vi "BilinearInterpolation.vi"(1 "Column Index":dbl, 2 "Row Index":dbl, 3 "Array":dbl[][](array[numeric])) -> (0 "Bilinear Interpolated Value":dbl)   [LabVIEW 2012]
uses:
  <vilib>/Analysis/baseanly.llb/Real Outer Product.vi
  <vilib>/Analysis/NI_AALBase.lvlib
panel:
  # "Bilinear Interpolation of a 2D array\n\n\nChristian Altenbach, June 2005\ncaltenba@ucla.edu"
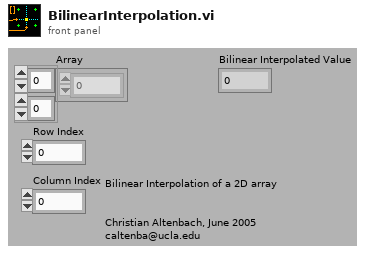
[diagram p1: front panel]
types:
  T1 = typedef "NI_Matrix.lvlib/RealMatrix.ctl" = dbl[][]
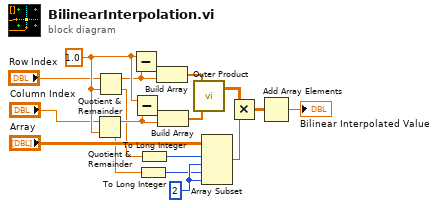
[diagram p0: block diagram]
diagram:
  w12 = 1.0 ("x")
  w18 = 2 ("length")
  n1 = Quotient & Remainder(x="Column Index", y=w12) -> (x-y*floor(x/y)=w7:dbl, floor(x/y)=w2:dbl)
  n2 = Quotient & Remainder(x="Row Index", y=w12) -> (x-y*floor(x/y)=w9:dbl, floor(x/y)=w3:dbl)
  n3 = Subtract(x=w12, y=w9) -> (x-y=w8:dbl)
  n4 = Subtract(x=w12, y=w7) -> (x-y=w6:dbl)
  n5 = To Long Integer(number=w2) -> (32bit integer=w14:i32)
  n6 = To Long Integer(number=w3) -> (32bit integer=w15:i32)
  n7 = Build Array(w8, w9) -> (w10:dbl[])
  n8 = Build Array(w6, w7) -> (w11:dbl[])
  n9 = call-poly <vilib>:"Outer Product.vi"("Y Vector"=w11, "X Vector"=w10) -> ("Outer Product"=w1:T1)  [unwired: 1 out]
  n10 = Array Subset(array="Array", index (row)=w15, length (row)=w18, index (col)=w14, length (col)=w18) -> (w13:dbl[][])
  n11 = Multiply(x=w1, y=w13) -> (x*y=w16:T1)
  n12 = Add Array Elements(numeric array=w16) -> (sum=→"Bilinear Interpolated Value":dbl)
